vi "Lockin.Create Low Pass Filter (FGV).vi"(6 "fs (Hz)":dbl, 7 "init [F]":bool, 8 "error in (no error)":errorcluster, 9 "Low Pass Cutoff (Hz)":dbl, 11 "order":i32=2) -> (0 "error out":errorcluster, 3 "Filters out":T1[](array[typedef]) {"mSRate_QSettings"."source" items=["Coef a/k"=0, "Coef b/v"=7, "Input"=1, "Output"=2, "Multiplicand"=3, "Product"=4, "Sum"=5, "Delay"=6, "Gain"=8]}, 5 "init out":bool)   [LabVIEW 2019, in "DSP.lvclass"]
uses:
  DSP.lvclass
  <vilib>/addons/Digital Filter Design/_Objects.llb/DFD Filter Obj.ctl
  <vilib>/addons/Digital Filter Design/_Objects.llb/DFD Filter Coef.ctl
  <vilib>/addons/Digital Filter Design/_Objects.llb/DFD Filter Structure Type Selector.ctl
  <vilib>/addons/Digital Filter Design/_Objects.llb/dfd_Internal Quantization Settings.ctl
  <vilib>/addons/Digital Filter Design/_Objects.llb/dfd_Internal Quantization Srcs.ctl
  <vilib>/addons/Digital Filter Design/_Objects.llb/DFD Coef Norm Type.ctl
  <vilib>/addons/Digital Filter Design/NI_DigFilterLicensed.lvlib
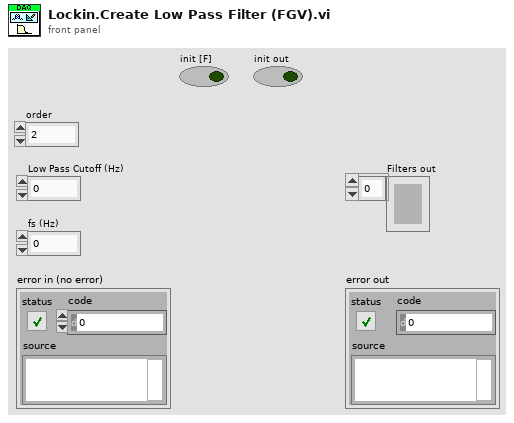
[diagram p1: front panel]
types:
  T1 = typedef "NI_DigFilterLicensed.lvlib/DFD Filter Obj.ctl" = cluster{"mSRate_Fs":dbl, "mSRate_Version":string, "mSRate_Comments":string, "mSRate_OrgCoef":T2, "mSRate_CurCoef":T2, "mSRate_Quantized?":bool, "mSRate_QCoef":T2, "mSRate_QSettings":T4[], "mSRate_Order":i32, "mSRate_Scaling":cluster{"mSRate_ScaleByPowerOf2?":bool, "mSRate_ScaleType":T6}}
  T2 = typedef "NI_DigFilterLicensed.lvlib/DFD Filter Coef.ctl" = cluster{"type":T3, "gain":dbl, "coef a (k)":dbl[], "coef b (v)":dbl[]}
  T3 = typedef "NI_DigFilterLicensed.lvlib/DFD Filter Structure Type Selector.ctl" = enum16{"Undefined", "FIR Direct Form", "FIR Direct Form Transposed", "FIR Symmetric", "FIR Antisymmetric", "IIR Direct Form I", "IIR Direct Form I Transposed", "IIR Direct Form II", "IIR Direct Form II Transposed", "IIR Cascaded Second Order Sections Form I", "IIR Cascaded Second Order Sections Form I Transposed", "IIR Cascaded Second Order Sections Form II", "IIR Cascaded Second Order Sections Form II Transposed", "Lattice Allpass (basic sections)", "Lattice Allpass (one multiplier sections)", "Lattice Allpass (normalized sections)", "Lattice AR (basic sections)", "Lattice AR (one multiplier sections)", "Lattice AR (normalized sections)", "Lattice MA (minimum phase)", "Lattice MA (maximum phase)", "Lattice ARMA (basic sections)", "Lattice ARMA (one multiplier sections)", "Lattice ARMA (normalized sections)"}
  T4 = typedef "NI_DigFilterLicensed.lvlib/dfd_Internal Quantization Settings.ctl" = cluster{"source":T5, "wl":i16, "iwl":i16, "overflow mode":enum16{"Saturation", "Wrap"}, "rounding mode":enum16{"Nearest", "Truncation"}, "signed?":bool}
  T5 = typedef "NI_DigFilterLicensed.lvlib/dfd_Internal Quantization Srcs.ctl" = u16
  T6 = typedef "NI_DigFilterLicensed.lvlib/DFD Coef Norm Type.ctl" = enum16{"No Norm", "Time Domain 1-Norm", "Time Domain 2-Norm", "Time Domain Inf-Norm"}
  T7 = enum16{"Lowpass", "Highpass", "Bandpass", "Bandstop"}
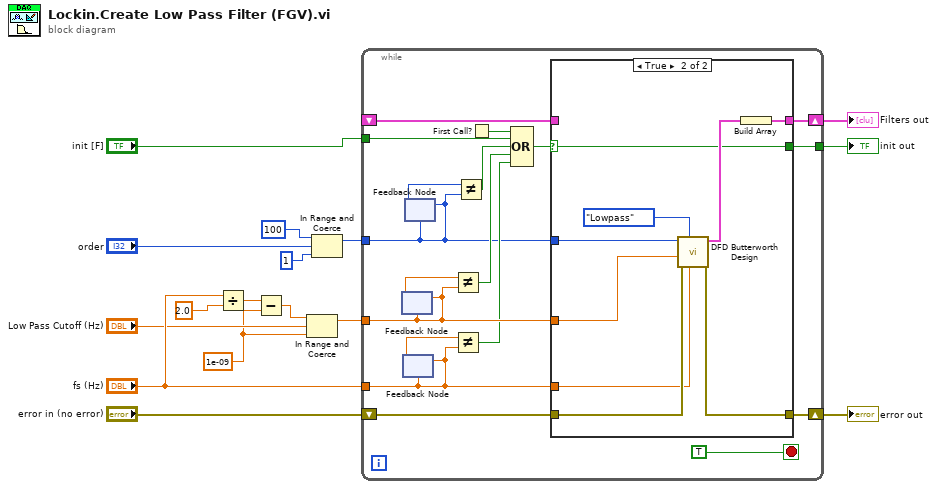
[diagram p0: block diagram]
diagram:
  w1 = 1e-09 ("lower limit")
  n1 = Divide(x="fs (Hz)", y=2.0 ("lower limit")) -> (x/y=w13:dbl)
  n2 = Subtract(x=w13, y=w1) -> (x-y=w12:dbl)
  n3 = In Range and Coerce(upper limit=w12, x="Low Pass Cutoff (Hz)", lower limit=w1) -> (coerced(x)=w8:dbl)  [unwired: 1 out]
  n4 = In Range and Coerce(upper limit=100, x="order", lower limit=1) -> (coerced(x)=w4:i32)  [unwired: 1 out]
  n5 = while {
    tunnel: w8 -> [w23]
    tunnel: "fs (Hz)" -> [w26]
    shift-right: [w32] -> w15
    shift-left: "error in (no error)" -> [w33]
    shift-right: [w34] -> w16
    shift-left: _ -> [w29]
    tunnel: "init [F]" -> [w28]
    tunnel: w4 -> [w19]
    tunnel: [w17] -> w2
    stop <- TRUE stop-if-true
    n6 = feedback #1(w23) -> (w24:dbl)
    n7 = feedback-in #1(w23) -> ()
    n8 = feedback #2(w26) -> (w25:dbl)
    n9 = feedback-in #2(w26) -> ()
    n10 = feedback #3(w19) -> (w22:i32)
    n11 = feedback-in #3(w19) -> ()
    n12 = Not Equal?(x=w24, y=w23) -> (x != y?=w30:bool)
    n13 = Not Equal?(x=w25, y=w26) -> (x != y?=w21:bool)
    n14 = Not Equal?(x=w22, y=w19) -> (x != y?=w20:bool)
    n15 = First Call?() -> (First Call?: T/F=w18:bool)
    n16 = Compound Arithmetic op=OR(w18, w28, w20, w30, w21) -> (w27:bool)
    n17 = case shown="True" w27 {
      selector: w27 -> [w35 w38]
      tunnel: [w37 w41] -> w34
      tunnel: w33 -> [w36 w45]
      tunnel: [w36 w44] -> w32
      tunnel: w23 -> [_ w40]
      tunnel: w26 -> [_ w43]
      tunnel: w29 -> [w37 _]
      tunnel: w19 -> [_ w39]
      tunnel: [w35 w38] -> w17
      frame False {
      }
      frame True {
        n18 = call <vilib>:"DFD Butterworth Design.vi"("fs [Hz]"=w43, "filter type"=T7."Lowpass", "error in (no error)"=w45, "low cutoff freq [Hz]"=w40, "order"=w39) -> ("error out"=w44:errorcluster, "filter out"=w42:T1)  [unwired: 5 in]
        n19 = Build Array(w42) -> (w41:T1[])
      }
    }
  }
  "init out" <- w2
  "Filters out" <- w16
  "error out" <- w15
